vi "UDP Tx Process.vi"(10 "Parameters":variant, 11 "Process":refnum<class "Process.lvclass">) -> ()   [LabVIEW 2016, in "UDP-Custom-Device Engine.lvlib"]
uses:
  UDP-Custom-Device Engine.lvlib
  <vilib>/NI/NIVS Inline Async API/_VS Inline Async API/Process/Process.lvclass
  <vilib>/NI/NIVS Inline Async API/_VS Inline Async API/Process/Process.lvclass/Process.ctl
  <vilib>/NI/NIVS Inline Async API/_Data Access Engine/Access Type Classes/Read/Read.lvclass/Read.ctl
  <vilib>/NI/NIVS Inline Async API/_Data Access Engine/Data Access Engine/Methods/Read.Data.vi
  <vilib>/NI/NIVS Inline Async API/_VS Inline Async API/Process/Data Member Access/Read Data Access.vi
  <vilib>/NI/NIVS Inline Async API/_VS Inline Async API/Error Handling Process/SubVIs/Error.ConvertArray.vi
  <vilib>/NI/NIVS Inline Async API/_Data Access Engine/Access Type Classes/Read/Read.ProcessData.vi
  <vilib>/NI/NIVS Inline Async API/_Data Access Engine/Data Access Engine/Data Access Engine.lvclass
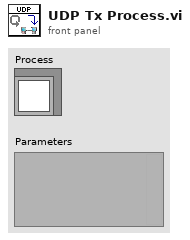
[diagram p1: front panel]
types:
  T1 = typedef "UDP-Custom-Device Engine.lvlib/Tx Loop Data.ctl" = cluster{"Packet Name":string, "Packet ID":i32, "Loop Period":u32, "Destination IP Address":string, "Destination Port":i32, "Tx FIFO Ref":T2, "Connection ID":refnum<k16>, "Local IP Address":string, "Local Port":i32, "Byte Order":enum16{"big-endian, network order", "native, host order", "little-endian"}, "Diagnostics En?":bool, "Header Info":bool[]}
  T2 = typedef "Data Access Engine.lvlib/Data Access Engine.lvclass/Read.DVR.ctl" = refnum<data-value>
  T3 = enum16{"big-endian, network order", "native, host order", "little-endian"}
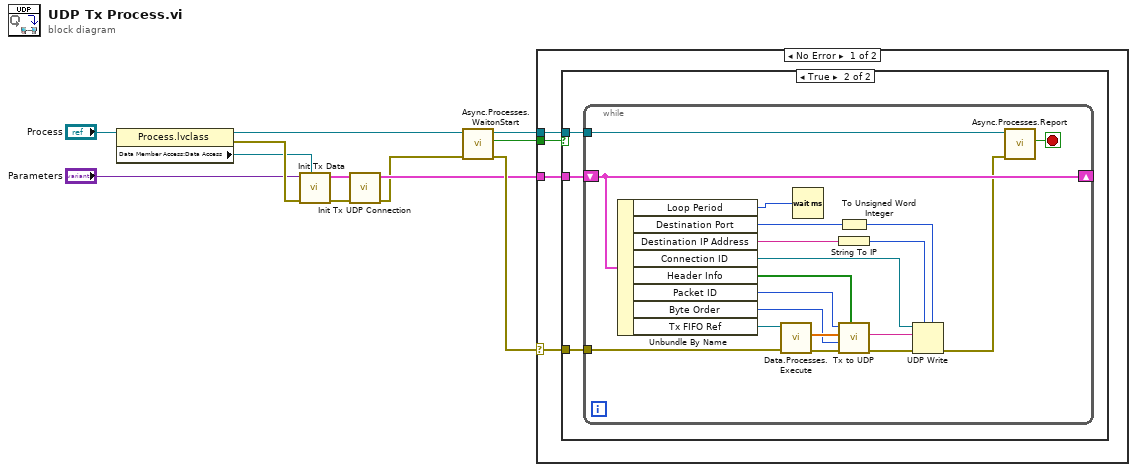
[diagram p0: block diagram]
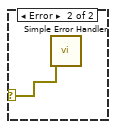
[diagram p3: hidden frame]
diagram:
  n1 = property class="Process.lvclass"(reference="Process") -> (reference out=w12:refnum<class "Process.lvclass">, error out=w6:errorcluster, "Data Member Access:Data Access"=w2:refnum<class "Data Access Engine.lvclass">)  [unwired: 1 in]
  n2 = call "Init Tx Data.vi"("Data Access in"=w2, "error in (no error)"=w6, "Parameters"="Parameters") -> ("error out"=w7:errorcluster, "Tx Loop Data"=w1:T1)  [unwired: 6 in, 1 out]
  n3 = call "Init Tx UDP Connection.vi"("error in (no error)"=w7, "Tx Loop Data in"=w1) -> ("error out"=w3:errorcluster, "Tx Loop Data out"=w4:T1)  [unwired: 8 in]
  n4 = call <vilib>:"Async.Processes.WaitonStart.vi"("error in (no error)"=w3, "Process"=w12) -> ("error out"=w10:errorcluster, "Execute"=w8:bool, "Process out"=w9:refnum<class "Process.lvclass">)  [unwired: 7 in]
  n5 = case shown="No Error" w10 {
    selector: w10 -> [w14 w39]
    tunnel: w8 -> [w16 _]
    tunnel: w9 -> [w15 _]
    tunnel: w4 -> [w13 _]
    frame No Error {
      n6 = case shown="True" w16 {
        tunnel: w14 -> [_ w18]
        tunnel: w15 -> [_ w19]
        tunnel: w13 -> [_ w17]
        frame False {
        }
        frame True {
          n7 = while {
            tunnel: w18 -> [w35]
            tunnel: w19 -> [w38]
            shift-right: [w36] -> _
            shift-left: w17 -> [w36]
            stop <- w37 stop-if-true
            n8 = Unbundle By Name(w36) -> ("Loop Period"=w20:u32, "Destination Port"=w29:i32, "Destination IP Address"=w22:string, "Connection ID"=w31:refnum<k16>, "Header Info"=w27:bool[], "Packet ID"=w24:i32, "Byte Order"=w25:T3, "Tx FIFO Ref"=w26:T2)
            n9 = call-poly <vilib>:"Data.Processes.Execute.vi"("error in (no error)"=w35, "Ref"=w26) -> ("error out"=w34:errorcluster, "Values"=w33:dbl[])  [unwired: 7 in, 1 out]
            n10 = Wait (ms)(milliseconds to wait=w20) -> ()  [unwired: 1 out]
            n11 = To Unsigned Word Integer(number=w29) -> (unsigned 16bit integer=w21:u16)
            n12 = String To IP(1:w22) -> (0:w30:u32)
            n13 = call "Tx to UDP.vi"("Header Info"=w27, "error in (no error)"=w34, "Byte Order"=w25, "Tx Array"=w33, "Packet ID"=w24) -> ("error out"=w32:errorcluster, "Tx String"=w23:string)  [unwired: 5 in]
            n14 = UDP Write(address=w30, port or service name=w21, connection ID=w31, data in=w23, 8:w32) -> (error out=w28:errorcluster)  [unwired: 1 in, 1 out]
            n15 = call <vilib>:"Async.Processes.Report.vi"("Error"=w28, "Process in"=w38) -> ("Stop"=w37:bool)  [unwired: 8 in, 1 out]
          }
        }
      }
    }
    frame Error {
      n16 = call <vilib>:"Simple Error Handler.vi"("error in (no error)"=w39) -> ()  [unwired: 4 in, 5 out]
    }
  }
